vi "Verify as JSON.vi"(5 "Options":T1, 7 "Test VI (caller)":string, 8 "error in":errorcluster, 10 "Anything":variant) -> (0 "error out":errorcluster, 1 "Failure Message":string, 2 "Passed?":bool)   [LabVIEW 2020, in "Approval Tests.lvlib"]
uses:
  Approval Tests.lvlib
  Options.ctl
  Reporter/Reporter.lvclass
  Printer/Printer.lvclass
  JSON Printer/JSON Printer.lvclass
  C:/Users/SAS/Desktop/approval-testing/Approval Tests/Printer/Printer.lvclass
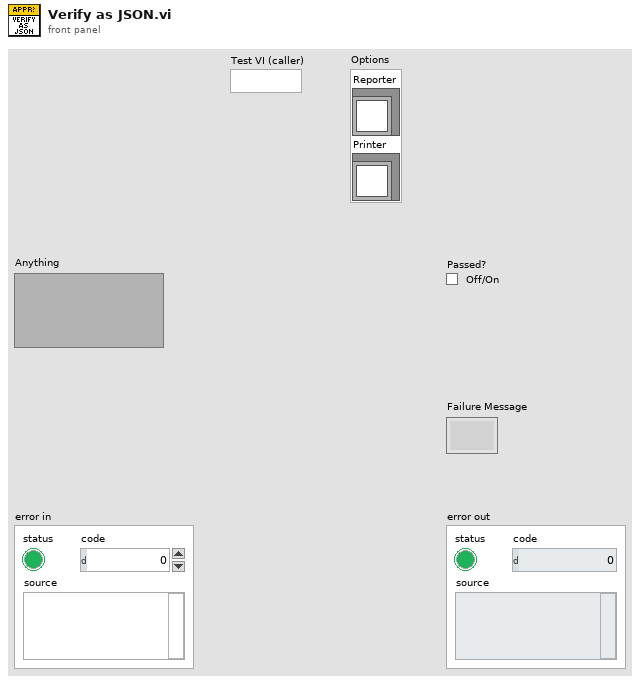
[diagram p1: front panel]
types:
  T1 = typedef "Approval Tests.lvlib/Options.ctl" = cluster{"Reporter":refnum<class "Reporter.lvclass">, "Printer":refnum<class "Printer.lvclass">}
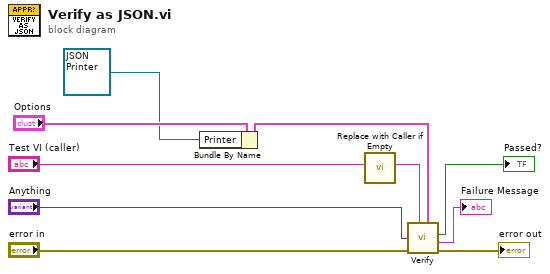
[diagram p0: block diagram]
diagram:
  n1 = Bundle By Name(cluster="Options", "Printer"=refnum<class "JSON Printer.lvclass"> refnum ("Approval Tests.lvlib:JSON Printer.lvclass")) -> (w3:T1)
  n2 = call "Replace with Caller if Empty.vi"("Test VI (caller) in"="Test VI (caller)") -> ("Test VI (caller) out"=w5:string)  [unwired: 10 in]
  n3 = call "Verify.vi"("Options"=w3, "Test VI (caller)"=w5, "error in"="error in", "Anything"="Anything") -> ("error out"=→"error out":errorcluster, "Failure Message"=→"Failure Message":string, "Passed?"=→"Passed?":bool)  [unwired: 5 in]
